vi "reading.vi"() -> ()   [LabVIEW 2014]
uses:
  <vilib>/Utility/error.llb/DialogType.ctl
  <vilib>/DAQmx/read.llb/DAQmx Read (Analog DBL 1Chan 1Samp).vi
  <vilib>/DAQmx/create/channels.llb/DAQmx Create Channel (AI-Voltage-Basic).vi
  <vilib>/DAQmx/configure/timing.llb/DAQmx Timing (Sample Clock).vi
  <vilib>/DAQmx/miscellaneous.llb/DAQmx Fill In Error Info.vi
panel:
  out "Array":u32[](array[numeric])
  out "Waveform Graph":dbl[](graph)
  out "Numeric":i32
  in  "Stop":bool
  out "Waveform Chart":dbl(graph)
  out "output array":dbl[](array[numeric])
  in  "Number of Samples":i32=100
  in  "Sample Rate":dbl=1000.0
  in  "Sample Clock Source":tag="OnboardClock"
  in  "Terminal Configuration":i32(ring)=-1 items=["default"=-1, "RSE"=10083, "NRSE"=10078, "Differential"=10106, "Pseudodifferential"=12529]
  in  "Max Voltage":dbl=5.0
  in  "Min Voltage":dbl=-5.0
  in  "Physical Channel":tag="Dev1/ai0"
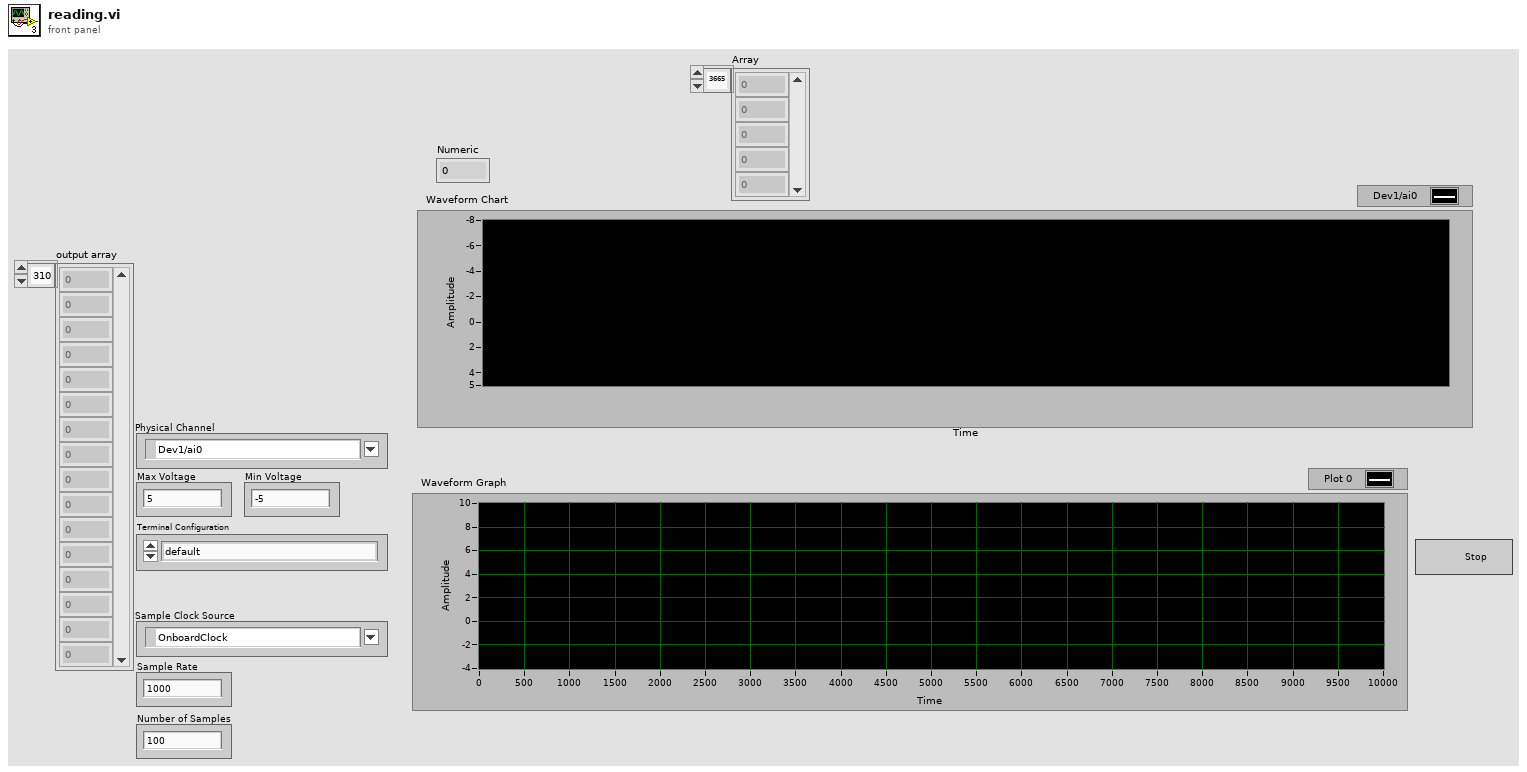
[diagram p1: front panel]
types:
  T1 = typedef "DialogType.ctl" = u16
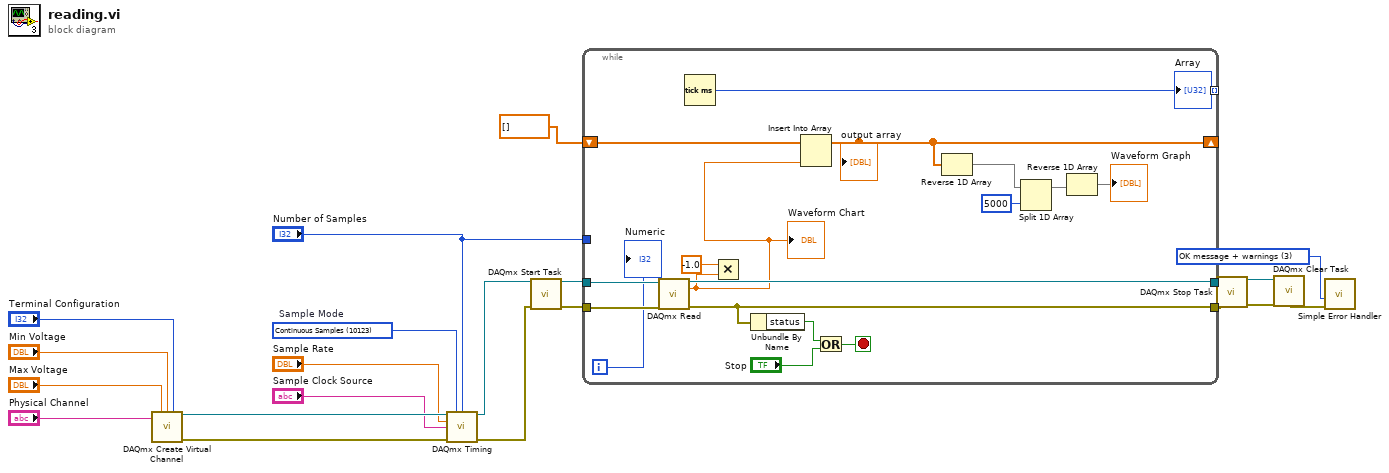
[diagram p0: block diagram]
diagram:
  w6 = T1 3 items=["no dialog", "OK message", "continue or stop message", "OK message + warnings", "continue/stop + warnings"] ("type of dialog (OK msg:1)")
  w22 = 10123 items=["Finite Samples"=10178, "Continuous Samples"=10123, "Hardware Timed Single Point"=12522]  # Sample Mode
  n1 = call-poly <vilib>:"DAQmx Create Virtual Channel.vi"("maximum value"="Max Voltage", "minimum value"="Min Voltage", "input terminal configuration"="Terminal Configuration", "physical channels"="Physical Channel") -> ("task out"=w20:refnum<k21>, "error out"=w21:errorcluster)  [unwired: 10 in]
  n2 = call-poly <vilib>:"DAQmx Timing.vi"("task/channels in"=w20, "sample mode"=w22, "samples per channel"="Number of Samples", "rate"="Sample Rate", "source"="Sample Clock Source", "error in"=w21) -> ("task out"=w4:refnum<k21>, "error out"=w3:errorcluster)  [unwired: 8 in]
  n3 = call <vilib>:"DAQmx Start Task.vi"("task/channels in"=w4, "error in"=w3) -> ("task out"=w13:refnum<k21>, "error out"=w12:errorcluster)  [unwired: 12 in]
  n4 = while {
    tunnel: w13 -> [w39]
    tunnel: w12 -> [w38]
    tunnel: [w37] -> w10
    tunnel: [w35] -> w9
    tunnel: "Number of Samples" -> [_]
    shift-right: [w26] -> _
    shift-left: dbl[] [] -> [w32]
    tunnel: [w30] -> w1 mode=indexing
    i -> [w31]
    stop <- w33 stop-if-true
    n5 = call-poly <vilib>:"DAQmx Read.vi"("task/channels in"=w39, "error in"=w38) -> ("task out"=w37:refnum<k21>, "data"=w23:dbl, "error out"=w35:errorcluster)  [unwired: 11 in]
    "Waveform Chart" <- w23
    n6 = Tick Count (ms)() -> (millisecond timer value=w30:u32)
    n7 = Multiply(x=-1.0, y=w23) -> ()  [unwired: 1 out]
    n8 = Unbundle By Name(w35) -> ("status"=w34:bool)
    n9 = Insert Into Array(array=w32, new element=w23) -> (w26:dbl[])  [unwired: 1 in]
    "output array" <- w26
    n10 = Or(x=w34, y="Stop") -> (x .or. y?=w33:bool)
    n11 = Reverse 1D Array(array=w26) -> (reversed array=w28:dbl[])
    n12 = Split 1D Array(array=w28, index=5000) -> (first subarray=w29:dbl[])  [unwired: 1 out]
    n13 = Reverse 1D Array(array=w29) -> (reversed array=→"Waveform Graph":dbl[])
    "Numeric" <- w31
  }
  "Array" <- w1
  n14 = call <vilib>:"DAQmx Stop Task.vi"("task/channels in"=w10, "error in"=w9) -> ("task out"=w7:refnum<k21>, "error out"=w8:errorcluster)  [unwired: 12 in]
  n15 = call <vilib>:"DAQmx Clear Task.vi"("task in"=w7, "error in"=w8) -> ("error out"=w11:errorcluster)  [unwired: 13 in]
  n16 = call <vilib>:"Simple Error Handler.vi"("type of dialog (OK msg:1)"=w6, "error in (no error)"=w11) -> ()  [unwired: 3 in, 5 out]
